vi "Passing Paramters Simple Struct.vi"(9 "radius":sgl, 10 "y":sgl, 11 "x":sgl) -> (3 "function return":sgl)   [LabVIEW 2018, in "ParsingDataSampleDLL.lvlib"]
doc: "__declspec(dllexport) float PassingParamters_SimpleStruct (struct simpleStructCircle circle);"
uses:
  ParsingDataSampleDLL.lvlib
  ni_reference_vs/Debug/ParsingDataSampleDLL.dll
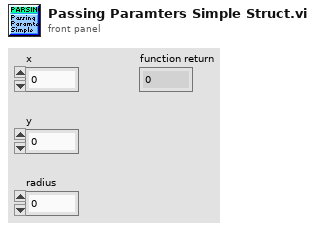
[diagram p1: front panel]
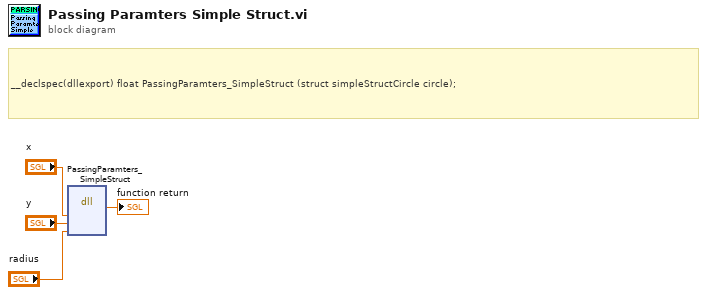
[diagram p0: block diagram]
diagram:
  # "__declspec(dllexport) float PassingParamters_SimpleStruct (struct simpleStructCircle circle);"
  n1 = dll-call lib="C:/Users/celit/Documents/GitHub/Labview_Python_DLL_Call/ni_reference_vs/Debug/ParsingDataSampleDLL.*" fn="PassingParamters_SimpleStruct"("x"="x", "y"="y", "radius"="radius") -> (→"function return":sgl)  [unwired: 6 in, 2 out]
